vi "Close_Instr.vi"(8 "error in (no error)":errorcluster caption="entrée d'erreur (pas d'erreur)", 11 "Class Instrument Firebase en entrée":refnum<class "Class Instrument Firebase Altyor.lvclass">) -> (0 "error out":errorcluster caption="sortie d'erreur", 3 "Class Instrument Firebase en sortie":refnum<class "Class Instrument Firebase Altyor.lvclass">)   [LabVIEW 2020, in "Library Instrument & Equipement.lvlib" / "Library Instruments.lvlib" / "Class Instrument Firebase Altyor.lvclass"]
uses:
  Class Instrument Firebase Altyor.lvclass
  Class Instrument Firebase Altyor.lvclass/Class Instrument Firebase Altyor.ctl
  Firebase/Source/Firebase Altyor/Firebase Altyor.lvclass
  C:/Users/ngarcin/OneDrive - Altyor/Standard TB/Class/Firebase/Source/Firebase Driver/Firebase Driver.lvclass
  Instrument (Default)/Class Instrument (Default).lvclass
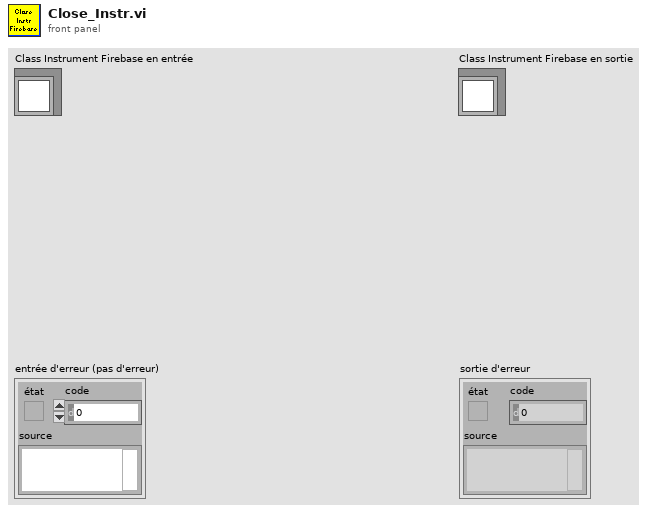
[diagram p1: front panel]
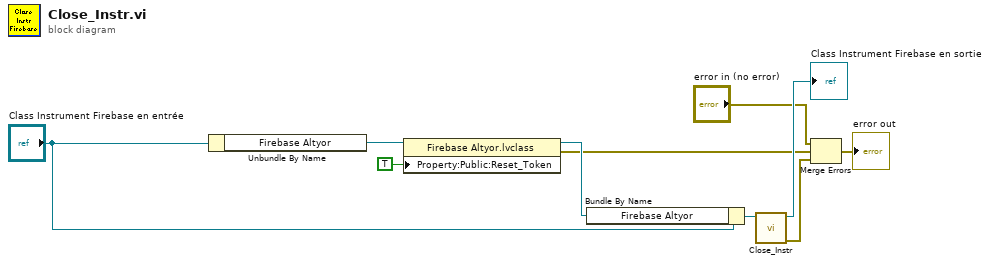
[diagram p0: block diagram]
diagram:
  n1 = Unbundle By Name("Class Instrument Firebase en entrée") -> ("Firebase Altyor"=w10:refnum<class "Firebase Altyor.lvclass">)
  n2 = property class="Firebase Altyor.lvclass"(reference=w10, "Property:Public:Reset_Token"=TRUE ("Reset_Token")) -> (reference out=w7:refnum<class "Firebase Altyor.lvclass">, error out=w3:errorcluster)  [unwired: 1 in]
  n3 = Bundle By Name(cluster="Class Instrument Firebase en entrée", "Firebase Altyor"=w7) -> (w5:refnum<class "Class Instrument Firebase Altyor.lvclass">)
  n4 = call-parent "Close_Instr.vi"("Class Instrument (Default) en entrée"=w5) -> ("error out"=w4:errorcluster, "Class Instrument (Default) en sortie"=→"Class Instrument Firebase en sortie":refnum<class "Class Instrument Firebase Altyor.lvclass">)  [unwired: 9 in]
  n5 = Merge Errors("error in (no error)", w3, w4) -> (→"error out":errorcluster)
